vi "Button Changed.vi"(11 "In":bool) -> (3 "button changed":bool)   [LabVIEW 2016]
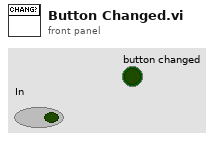
[diagram p1: front panel]
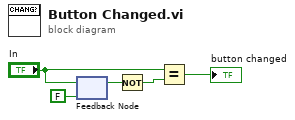
[diagram p0: block diagram]
diagram:
  n1 = feedback #1(FALSE) -> (w3:bool)
  n2 = feedback-in #1("In") -> ()
  n3 = Not(x=w3) -> (.not. x?=w4:bool)
  n4 = Equal?(x="In", y=w4) -> (x = y?=→"button changed":bool)
